vi "set gear information.vi"(8 "error in (no error)":errorcluster, 10 "gear_information":T1, 11 "id":i32) -> (0 "error out":errorcluster, 3 "function return":i32)   [LabVIEW 2012, in "libximc.lvlib"]
doc: "result_t XIMC_API set_gear_information (device_t id, const gear_information_t* gear_information);"
uses:
  libximc.lvlib
  libximc.dll
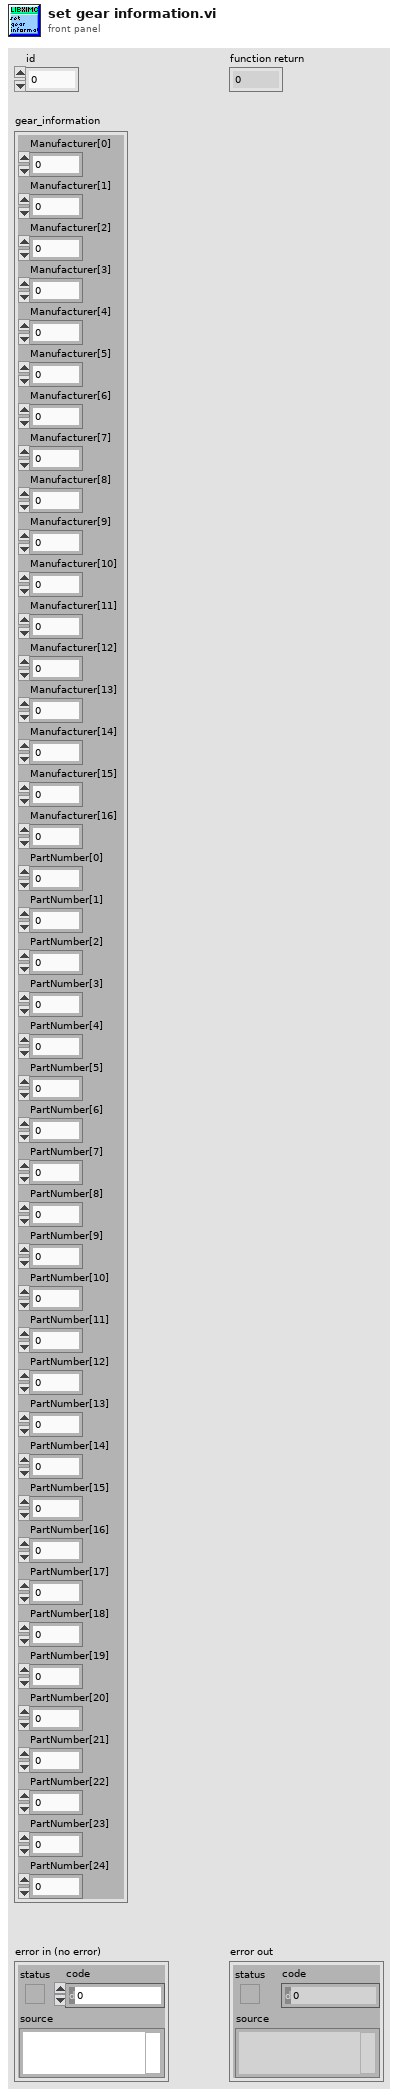
[diagram p1: front panel]
types:
  T1 = cluster{"Manufacturer[0]":i8, "Manufacturer[1]":i8, "Manufacturer[2]":i8, "Manufacturer[3]":i8, "Manufacturer[4]":i8, "Manufacturer[5]":i8, "Manufacturer[6]":i8, "Manufacturer[7]":i8, "Manufacturer[8]":i8, "Manufacturer[9]":i8, "Manufacturer[10]":i8, "Manufacturer[11]":i8, "Manufacturer[12]":i8, "Manufacturer[13]":i8, "Manufacturer[14]":i8, "Manufacturer[15]":i8, "Manufacturer[16]":i8, "PartNumber[0]":i8, "PartNumber[1]":i8, "PartNumber[2]":i8, "PartNumber[3]":i8, "PartNumber[4]":i8, "PartNumber[5]":i8, "PartNumber[6]":i8, "PartNumber[7]":i8, "PartNumber[8]":i8, "PartNumber[9]":i8, "PartNumber[10]":i8, "PartNumber[11]":i8, "PartNumber[12]":i8, "PartNumber[13]":i8, "PartNumber[14]":i8, "PartNumber[15]":i8, "PartNumber[16]":i8, "PartNumber[17]":i8, "PartNumber[18]":i8, "PartNumber[19]":i8, "PartNumber[20]":i8, "PartNumber[21]":i8, "PartNumber[22]":i8, "PartNumber[23]":i8, "PartNumber[24]":i8}
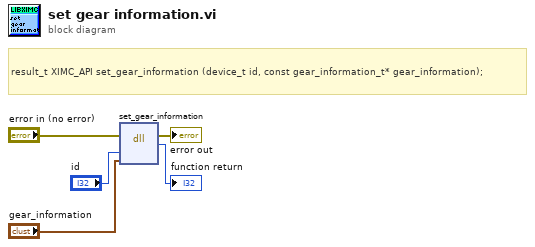
[diagram p0: block diagram]
diagram:
  # "result_t XIMC_API set_gear_information (device_t id, const gear_information_t* gear_information);"
  n1 = dll-call lib="C:/Users/Stepan/Downloads/labview_2.9.11_testgen_thread/libximc.*" fn="set_gear_information"(error in="error in (no error)", "id"="id", "gear_information"="gear_information") -> (error out=→"error out":errorcluster, →"function return":i32)  [unwired: 4 in, 1 out]
